vi "Gergberg v2.vi"() -> ()   [LabVIEW 2012, in "LightPipes.lvlib"]
uses:
  Lightpipes.lvlib
panel:
  out "Original Target":dbl[][](graph)
  out "Retrieved Target":dbl[][](graph)
  out "Target Intensity\n RMS Error":dbl(graph)
  in  "Target Final Beam":path=path "C:/Users/Tri Nguyen/Documents/lightpipes/LabView/beam images/target_retrieved.pgm"
  in  "size_grid":dbl=0.02
  in  "n_grid":i32=256
  in  "Target":path=path "C:/Users/Tri Nguyen/Documents/lightpipes/LabView/beam images/target_int.gpl"
  in  "Number of Iteration":i32=5
  out "Iteration":i32=4
  in  "Show Phase Iterations":bool=TRUE
  in  "Show Intensity Iterations":bool=TRUE
  out "Retrieved Target \nPhase Graph":dbl[][](graph)
  in  "Source":path=path "C:/Users/Tri Nguyen/Documents/lightpipes/LabView/beam images/initial_int.gpl"
  in  "PGM gamma":dbl=1.0
  in  "forward distance":dbl=0.5
  # "Beam Information"
  # "Iteration"
  # "Beam Intensity Files"
  # "Retrieved Files"
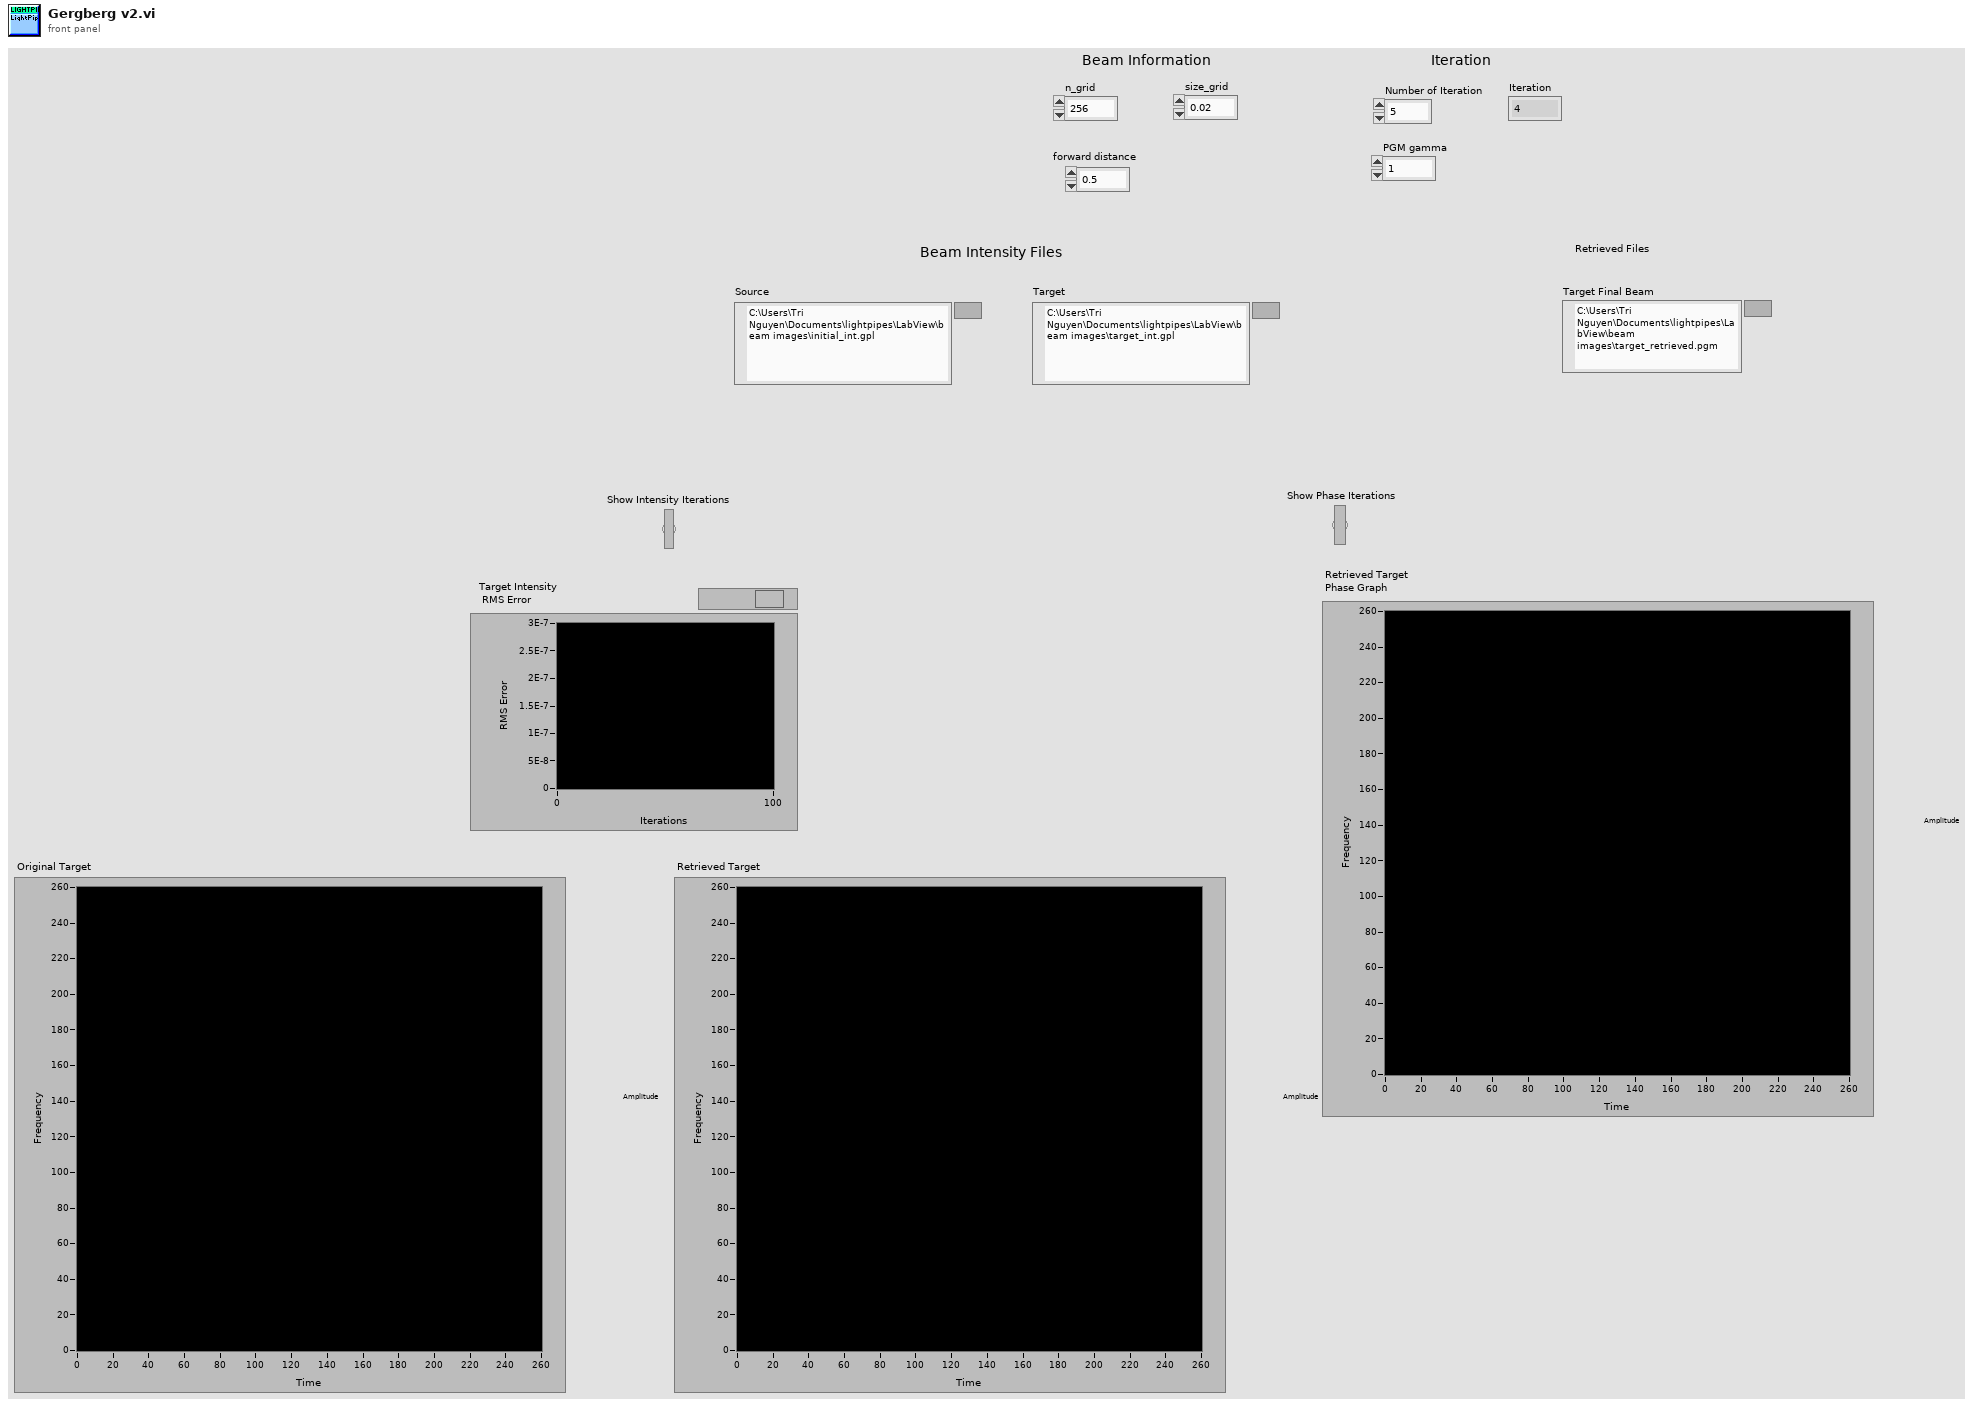
[diagram p1: front panel]
types:
  T1 = cluster{"n_grid":i32, "@dummy control@":i8, "@dummy control@":i8, "@dummy control@":i8, "@dummy control@":i8, "size":dbl, "lambda":dbl, "int1":i32, "int2":i32, "int3":i32, "@dummy control@":i8, "@dummy control@":i8, "@dummy control@":i8, "@dummy control@":i8, "double1":dbl, "double2":dbl, "double3":dbl, "real":u32, "imaginary":u32}
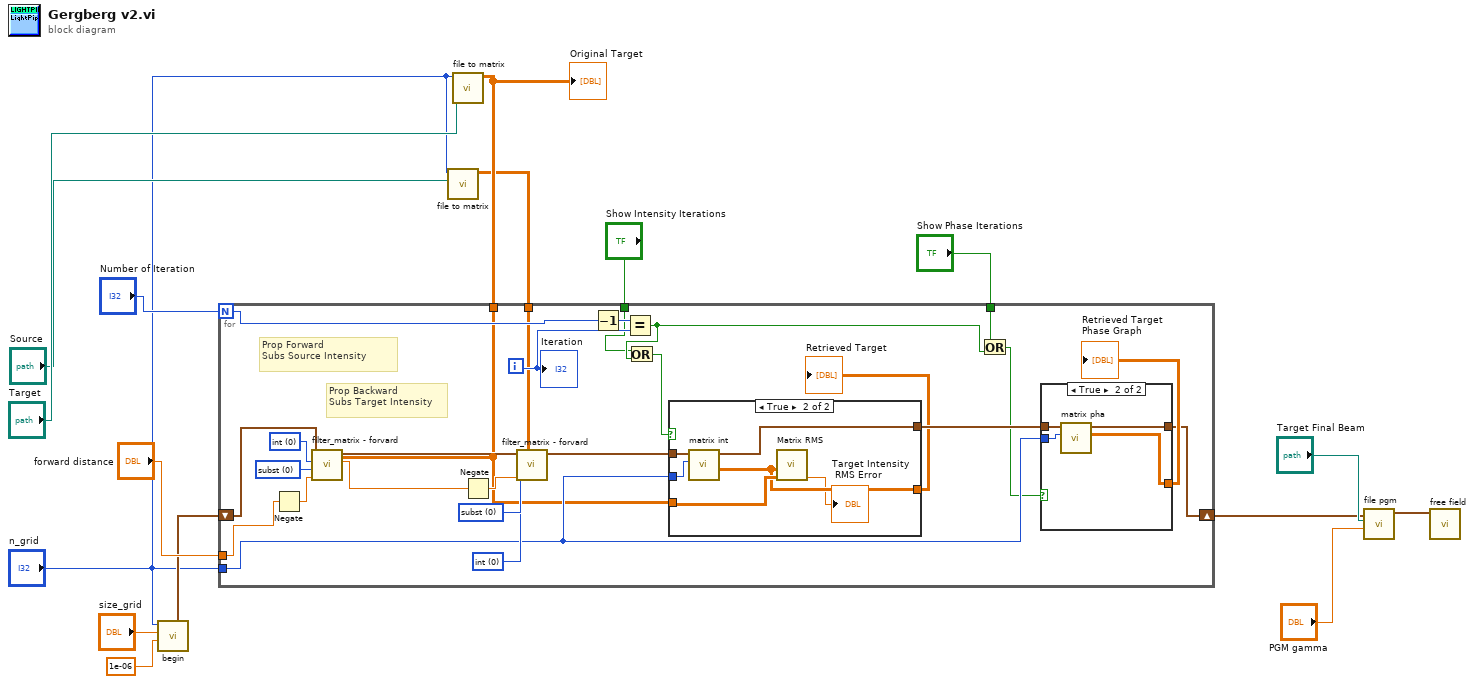
[diagram p0: block diagram]
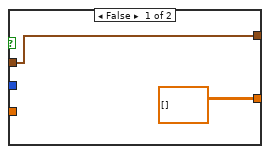
[diagram p2: hidden frame]
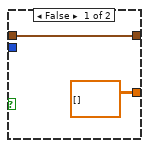
[diagram p3: hidden frame]
diagram:
  n1 = call "begin.vi"("lambda"=1e-06, "size_grid"="size_grid", "n_grid"="n_grid") -> ("field out"=w6:T1)  [unwired: 8 in]
  n2 = call "file to matrix.vi"("File Path"="Source", "number of rows (all:-1)"="n_grid") -> ("all rows"=w3:dbl[][])  [unwired: 9 in]
  n3 = call "file to matrix.vi"("File Path"="Target", "number of rows (all:-1)"="n_grid") -> ("all rows"=w5:dbl[][])  [unwired: 9 in]
  "Original Target" <- w5
  n4 = for {
    N: "Number of Iteration" -> [w30]
    shift-right: [w18] -> w8
    shift-left: w6 -> [w37]
    tunnel: "forward distance" -> [w36]
    tunnel: "n_grid" -> [w31]
    tunnel: "Show Intensity Iterations" -> [w24]
    tunnel: "Show Phase Iterations" -> [w23]
    tunnel: w5 -> [w17]
    tunnel: w3 -> [w19]
    i -> [w29]
    w39 = i16 0 items=["int", "pha"] ("intensity/phase")
    w40 = i16 0 items=["subst", "mult"] ("multiplication/substitution")
    w41 = i16 0 items=["int", "pha"] ("intensity/phase")
    w42 = i16 0 items=["subst", "mult"] ("multiplication/substitution")
    # "Prop Backward\nSubs Target Intensity"
    # "Prop Forward\nSubs Source Intensity"
    n5 = Negate(x=w36) -> (-x=w35:dbl)
    n6 = call "filter_matrix - forvard.vi"("matrix in"=w17, "forward distance"=w35, "multiplication/substitution"=w40, "intensity/phase"=w39, "field"=w37) -> ("forwarded dist"=w21:dbl, "field out"=w34:T1)  [unwired: 5 in]
    n7 = Negate(x=w21) -> (-x=w20:dbl)
    n8 = call "filter_matrix - forvard.vi"("matrix in"=w19, "forward distance"=w20, "multiplication/substitution"=w42, "intensity/phase"=w41, "field"=w34) -> ("field out"=w33:T1)  [unwired: 5 in, 1 out]
    n9 = Decrement(x=w30) -> (x-1=w28:i32)
    n10 = Equal?(x=w28, y=w29) -> (x = y?=w26:bool)
    n11 = Or(x=w24, y=w26) -> (x .or. y?=w27:bool)
    n12 = case shown="True" w27 {
      tunnel: [w44 w50] -> w38
      tunnel: w17 -> [_ w48]
      tunnel: w31 -> [_ w49]
      tunnel: w33 -> [w44 w47]
      tunnel: [dbl[][] [] ("matrix out 2D") w46] -> w22
      frame False {
      }
      frame True {
        n13 = call "matrix int.vi"("n_grid"=w49, "field"=w47) -> ("matrix out 2D"=w46:dbl[][], "field out"=w50:T1)  [unwired: 8 in]
        n14 = call "Matrix RMS.vi"("Original Matrix"=w48, "Iterative Matrix"=w46) -> ("RMS"=→"Target Intensity\n RMS Error":dbl)  [unwired: 9 in]
      }
    }
    "Retrieved Target" <- w22
    n15 = Or(x=w23, y=w26) -> (x .or. y?=w25:bool)
    n16 = case shown="True" w25 {
      tunnel: w38 -> [w52 w56]
      tunnel: [w52 w55] -> w18
      tunnel: w31 -> [_ w53]
      tunnel: [dbl[][] [] ("Phase") w54] -> w32
      frame False {
      }
      frame True {
        n17 = call "matrix pha.vi"("n_grid"=w53, "field"=w56) -> ("matrix out 2D"=w54:dbl[][], "field out"=w55:T1)  [unwired: 8 in]
      }
    }
    "Retrieved Target \nPhase Graph" <- w32
    "Iteration" <- w29
  }
  n18 = call "file pgm.vi"("gamma"="PGM gamma", "Path"="Target Final Beam", "field"=w8) -> ("field out"=w7:T1)  [unwired: 7 in, 1 out]
  n19 = call "free field.vi"("field"=w7) -> ()  [unwired: 10 in, 1 out]
